vi "MOpen.vi"(0 "Board":u8, 7 "error in (no error)":errorcluster) -> (10 "Handle 15":u32, 11 "Handle 16":u32, 12 "Handle 13":u32, 13 "Handle 14":u32, 14 "Handle 11":u32, 15 "Handle 12":u32, 16 "Handle 9":u32, 17 "Handle 10":u32, 18 "Handle 7":u32, 19 "Handle 8":u32, 20 "Status":i32, 21 "Handle 1":u32, 22 "Handle 2":u32, 23 "Handle 3":u32, 24 "Handle 4":u32, 25 "Handle 5":u32, 26 "Handle 6":u32, 27 "error out":errorcluster)   [LabVIEW 2016, in "Photon Counter.lvlib" / "C8855-01.lvlib"]
doc: "Resets the driver and acquires a handle to control this unit. Use this function when controlling two or more C8855-01 units.\n\n\nBOOL C8855API __stdcall C8855MOpen( BYTE board,\n HANDLE *hC8855_1,\n HANDLE *hC8855_2,\n HANDLE *hC8855_3,\n HANDLE *hC8855_4,\n HANDLE *hC8855_5,\n HANDLE *hC8855_6,\n HANDLE *hC8855_7,\n HANDLE *hC8855_8,\n HANDLE *hC8855_9,\n HANDLE *hC8855_10,\n HANDLE *hC8855_11,\n HANDLE *hC8855_12,\n HANDLE *hC8855_13,\n HANDLE *hC8855_14,\n HANDLE *hC8855_15,\n HANDLE *hC8855_16);"
uses:
  C8855-01.lvlib
  C8855-01api.dll
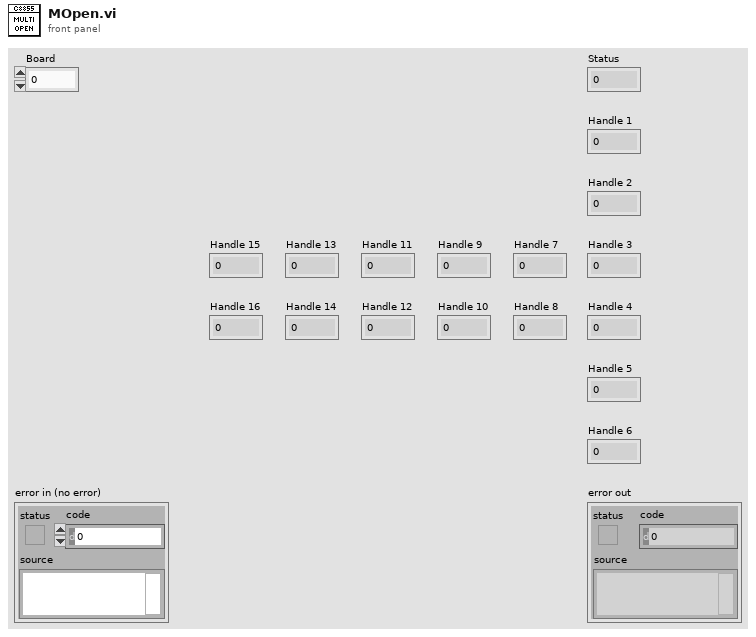
[diagram p1: front panel]
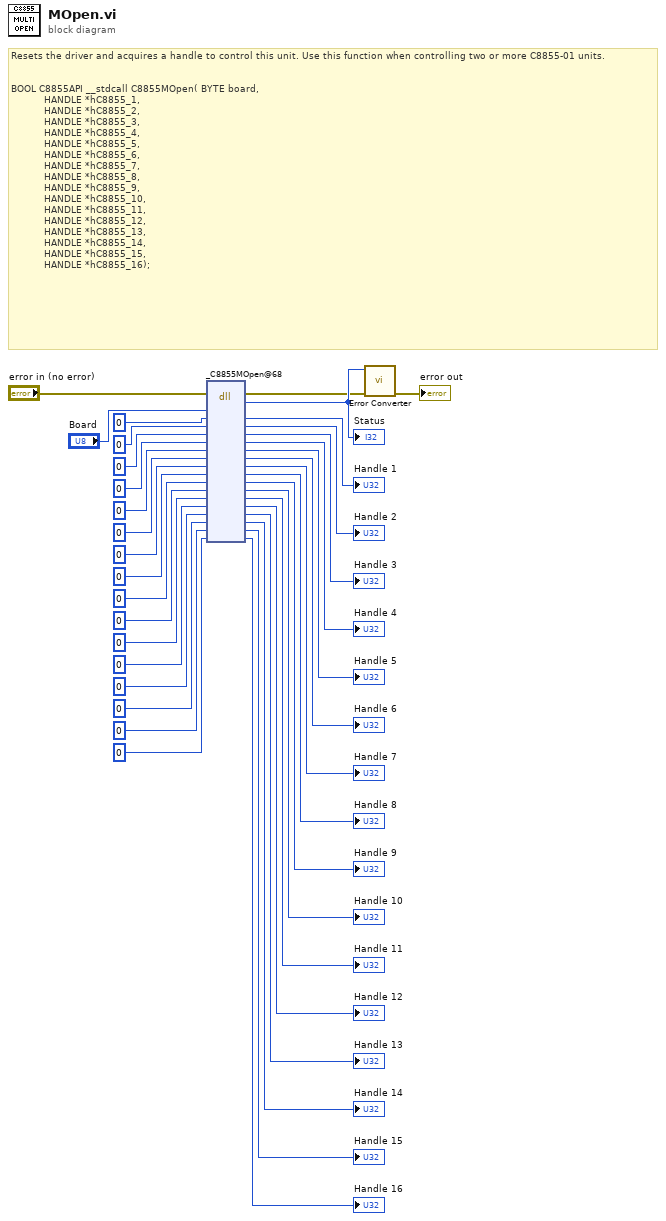
[diagram p0: block diagram]
diagram:
  # "Resets the driver and acquires a handle to control this unit. Use this function when controlling two or more C8855-01 units.\n\n\nBOOL C8855API __stdcall C8855MOpen( BYTE board,\n\t\t\t\t\t\t\t\t   HANDLE *hC8855_1,\n\t\t\t\t\t\t\t\t   HANDLE *hC8855_2,\n\t\t\t\t\t\t\t\t   HANDLE *hC8855_3,\n\t\t\t\t\t\t\t\t   HANDLE *hC8855_4,\n\t\t\t\t\t\t\t\t   HANDLE *hC8855_5,\n\t\t\t\t\t\t\t\t   HANDLE *hC8855_6,\n\t\t\t\t\t\t\t\t   HANDLE *hC8855_7,\n\t\t\t\t\t\t\t\t   HANDLE *hC8855_8,\n\t\t\t\t\t\t\t\t   HANDLE *hC8855_9,\n\t\t\t\t\t\t\t\t   HANDLE *hC8855_10,\n\t\t\t\t\t\t\t\t   HANDLE *hC8855_11,\n\t\t\t\t\t\t\t\t   HANDLE *hC8855_12,\n\t\t\t\t\t\t\t\t   HANDLE *hC8855_13,\n\t\t\t\t\t\t\t\t   HANDLE *hC8855_14,\n\t\t\t\t\t\t\t\t   HANDLE *hC8855_15,\n\t\t\t\t\t\t\t\t   HANDLE *hC8855_16);"
  n1 = dll-call lib="C:/Users/Andy/Desktop/Trace Grabber/Drivers/C8855-01/C8855-01api.*" fn="_C8855MOpen@68"(error in="error in (no error)", "Board"="Board", "Handle 1"=u32 0, "Handle 2"=u32 0, "Handle 3"=u32 0, "Handle 4"=u32 0, "Handle 5"=u32 0, "Handle 6"=u32 0, "Handle 7"=u32 0, "Handle 8"=u32 0, "Handle 9"=u32 0, "Handle 10"=u32 0, "Handle 11"=u32 0, "Handle 12"=u32 0, "Handle 13"=u32 0, "Handle 14"=u32 0, "Handle 15"=u32 0, "Handle 16"=u32 0) -> (error out=w2:errorcluster, w37:i32, "Handle 1"=→"Handle 1":u32, "Handle 2"=→"Handle 2":u32, "Handle 3"=→"Handle 3":u32, "Handle 4"=→"Handle 4":u32, "Handle 5"=→"Handle 5":u32, "Handle 6"=→"Handle 6":u32, "Handle 7"=→"Handle 7":u32, "Handle 8"=→"Handle 8":u32, "Handle 9"=→"Handle 9":u32, "Handle 10"=→"Handle 10":u32, "Handle 11"=→"Handle 11":u32, "Handle 12"=→"Handle 12":u32, "Handle 13"=→"Handle 13":u32, "Handle 14"=→"Handle 14":u32, "Handle 15"=→"Handle 15":u32, "Handle 16"=→"Handle 16":u32)  [unwired: 3 in, 1 out]
  "Status" <- w37
  n2 = call "Error Converter.vi"("error in (no error)"=w2, "error code"=w37) -> ("error out"=→"error out":errorcluster)  [unwired: 9 in]
